vi "Append Hypertext Link Anchor to Report.vi"(0 "report in":refnum<class "NI_Word.lvclass">, 1 "MS Office parameters":T1, 5 "URL of link - href":string, 9 "link text":string, 11 "error in (no error)":errorcluster) -> (4 "report out":refnum<class "NI_Word.lvclass">, 8 "start out (Word)":i32, 10 "end out (Word)":i32, 15 "error out":errorcluster)   [LabVIEW 2017, in "NI_Word.lvclass"]
doc: "Creates and adds a hypertext link anchor to a Word, Excel, or HTML report. You cannot use this VI with standard reports."
uses:
  <vilib>/Utility/NIReport.llb/Word/NI_Word.lvclass
  <vilib>/Utility/NIReport.llb/Word/NI_Word.lvclass/NI_Word.ctl
  <vilib>/addons/_office/NI_ReportGenerationToolkit.lvlib
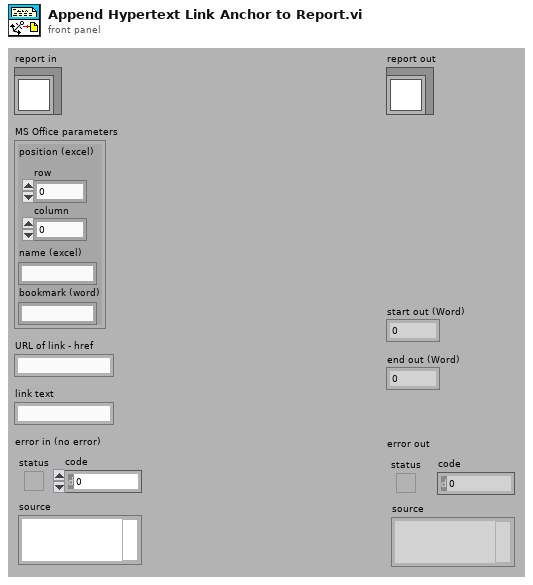
[diagram p1: front panel]
types:
  T1 = cluster{"position (excel)":cluster{"row":i32, "column":i32}, "name (excel)":string, "bookmark (word)":string}
  T2 = typedef "NI_ReportGenerationCore.lvlib/Report Data Members.ctl" = cluster{"font":T3, "from template?":bool}
  T3 = typedef "NI_ReportGenerationCore.lvlib/font.ctl" = cluster{"font name":string, "font size":dbl, "bold":u16, "italic":u16, "underline":u16, "strike through":u16, "font color":u32}
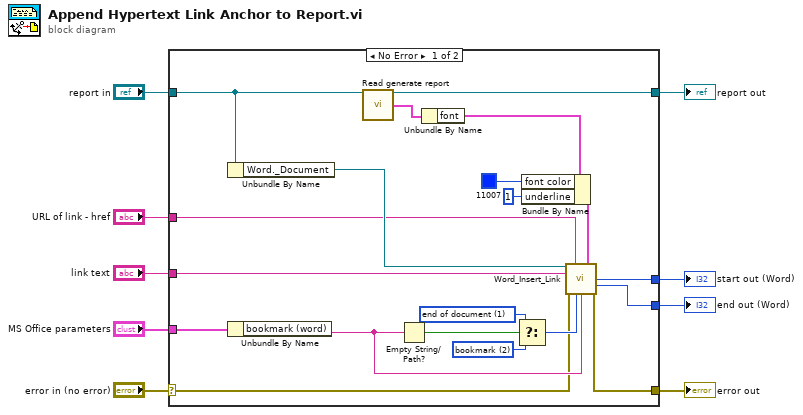
[diagram p0: block diagram]
diagram:
  n1 = case shown="No Error" "error in (no error)" {
    selector: "error in (no error)" -> [w20 w31]
    tunnel: [w19 w31] -> w8
    tunnel: [w12 w30] -> w6
    tunnel: "report in" -> [w13 w30]
    tunnel: "MS Office parameters" -> [w18 _]
    tunnel: "URL of link - href" -> [w17 _]
    tunnel: "link text" -> [w16 _]
    tunnel: [w15 _] -> w2
    tunnel: [w14 _] -> w1
    frame No Error {
      w23 = u16 2 items=["begining of document", "end of document", "bookmark", "custom"] ("Insertion point")
      w21 = u16 1 items=["begining of document", "end of document", "bookmark", "custom"] ("Insertion point")
      n2 = Unbundle By Name(w13) -> ("Word._Document"=w28:refnum<k7>)
      n3 = Unbundle By Name(w18) -> ("bookmark (word)"=w26:string)
      n4 = call-dynamic "Read generate report.vi"("report in"=w13) -> ("report out"=w12:refnum<class "NI_Word.lvclass">, "generate report"=w11:T2)  [unwired: 12 in, 1 out]
      n5 = Empty String/Path?(string/path=w26) -> (empty?=w22:bool)
      n6 = Unbundle By Name(w11) -> ("font"=w10:T3)
      n7 = Select(t=w21, s=w22, f=w23) -> (s? t:f=w27:u16)
      n8 = Bundle By Name(cluster=w10, "font color"=u32 11007, "underline"=u16 1) -> (w29:T3)
      n9 = call <vilib>:"Word_Insert_Link.vi"("Word._Document"=w28, "Address"=w17, "font"=w29, "Text to display"=w16, "Error in"=w20, "Insertion point"=w27, "bookmark name"=w26) -> ("Start out"=w15:i32, "End out"=w14:i32, "Error out"=w19:errorcluster)  [unwired: 3 in, 3 out]
    }
    frame Error {
    }
  }
  "error out" <- w8
  "report out" <- w6
  "start out (Word)" <- w2
  "end out (Word)" <- w1
